vi "Write DAQmx Device Name.vi"(8 "error in (no error)":errorcluster, 10 "DAQmx Device Name":tag, 11 "DAQmx Digitizer in":refnum<class "DAQmx Synthesizer.lvclass">) -> (0 "error out":errorcluster, 3 "DAQmx Digitizer out":refnum<class "DAQmx Synthesizer.lvclass">)   [LabVIEW 2019, in "DAQmx Synthesizer.lvclass"]
uses:
  DAQmx Synthesizer.lvclass
  DAQmx Synthesizer.lvclass/DAQmx Synthesizer.ctl
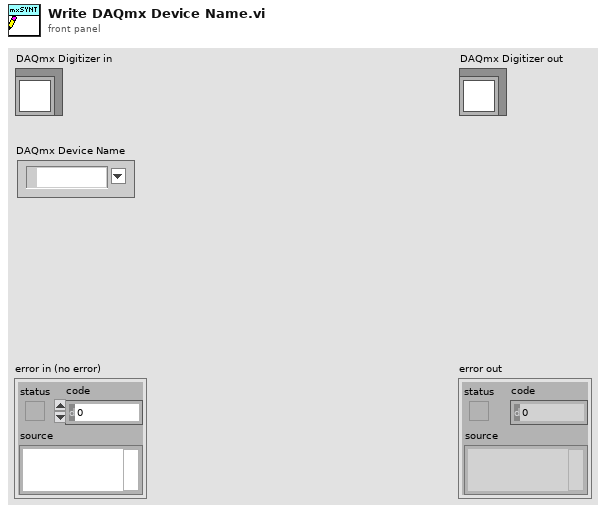
[diagram p1: front panel]
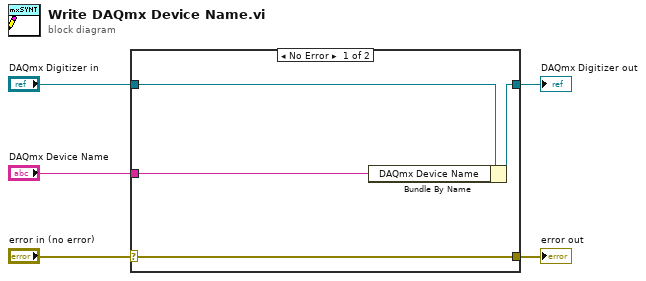
[diagram p0: block diagram]
diagram:
  n1 = case shown="No Error" "error in (no error)" {
    selector: "error in (no error)" -> [w9 w10]
    tunnel: [w9 w10] -> w4
    tunnel: [w7 w11] -> w2
    tunnel: "DAQmx Digitizer in" -> [w8 w11]
    tunnel: "DAQmx Device Name" -> [w6 _]
    frame No Error {
      n2 = Bundle By Name(cluster=w8, "DAQmx Device Name"=w6) -> (w7:refnum<class "DAQmx Synthesizer.lvclass">)
    }
    frame Error {
    }
  }
  "error out" <- w4
  "DAQmx Digitizer out" <- w2
